vi "Durability_will_2012_07_17_main_single_debug.vi"() -> ()   [LabVIEW 2011]
panel:
  out "error out":errorcluster
  in  "Speed 1":i8(slide)=50 min=0 max=100 step=10 scale=0.0..100.0
  in  "Quit 4":bool
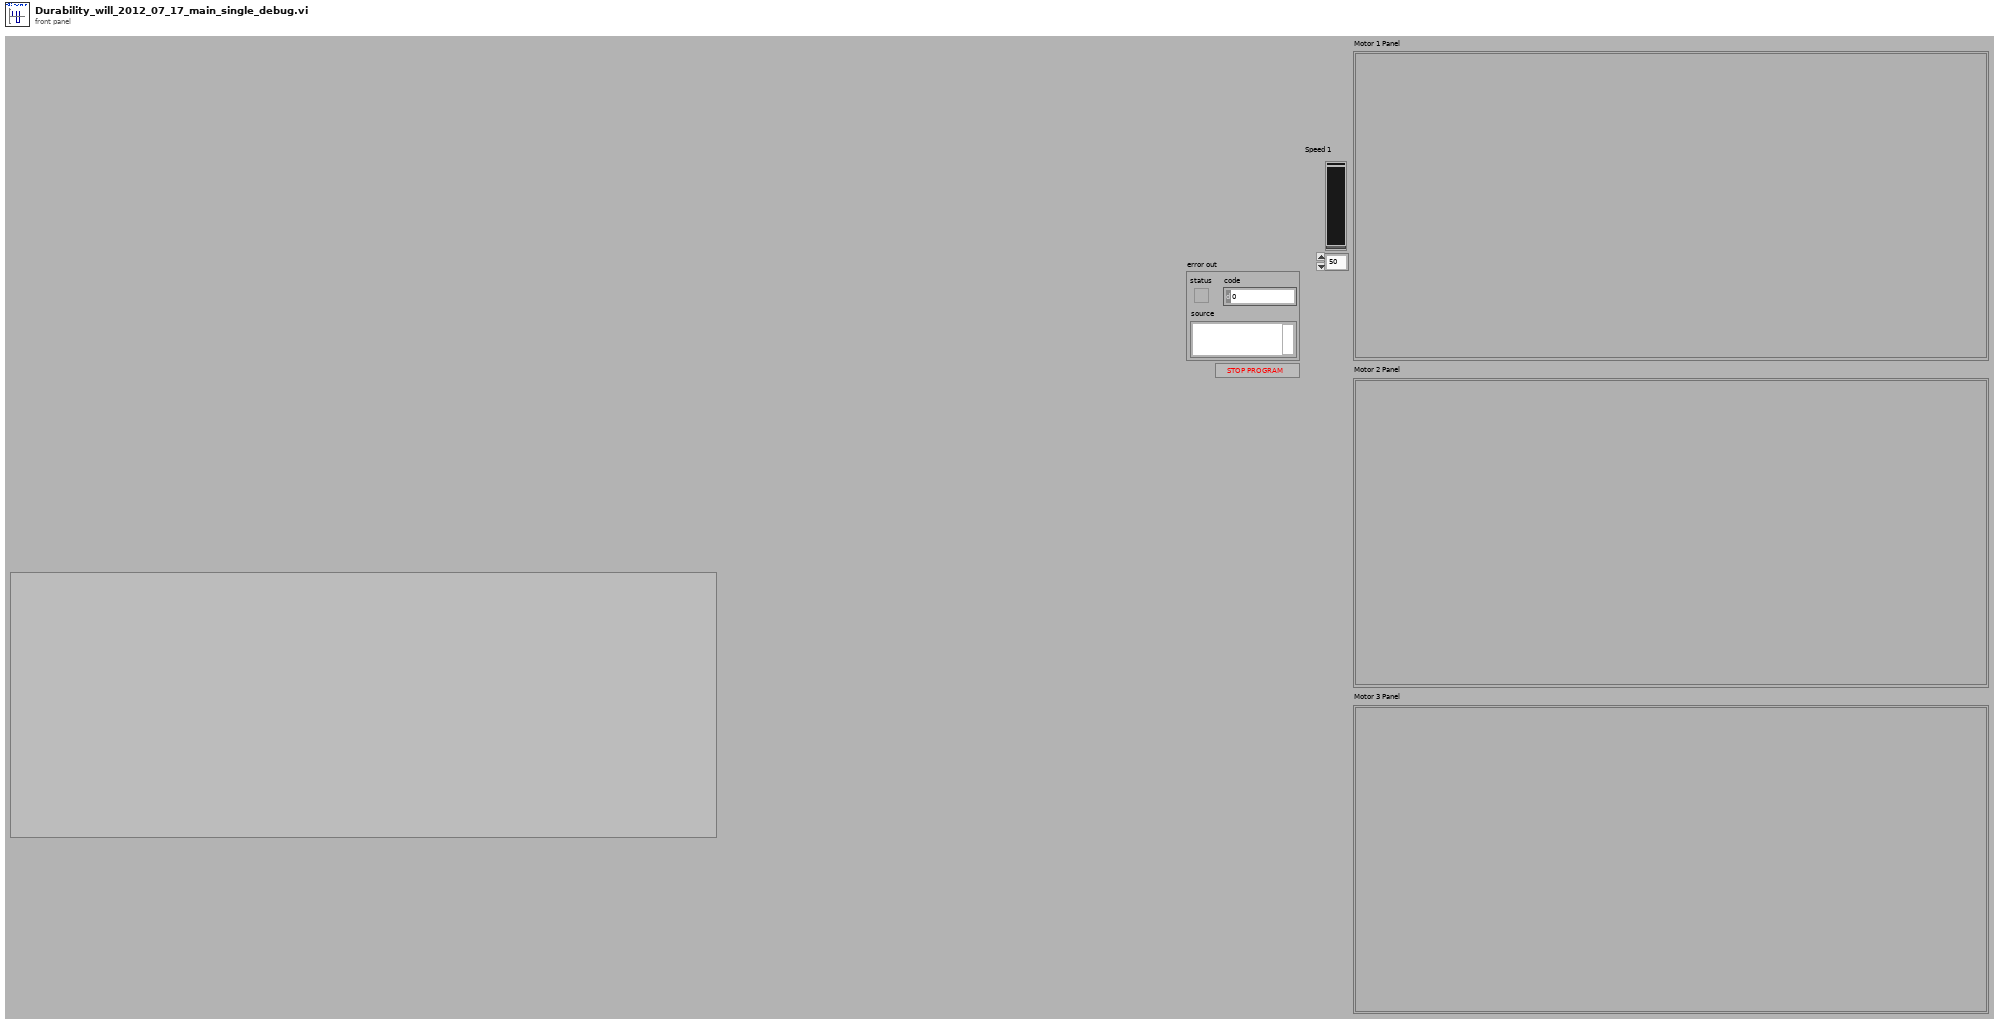
[diagram p1: front panel]
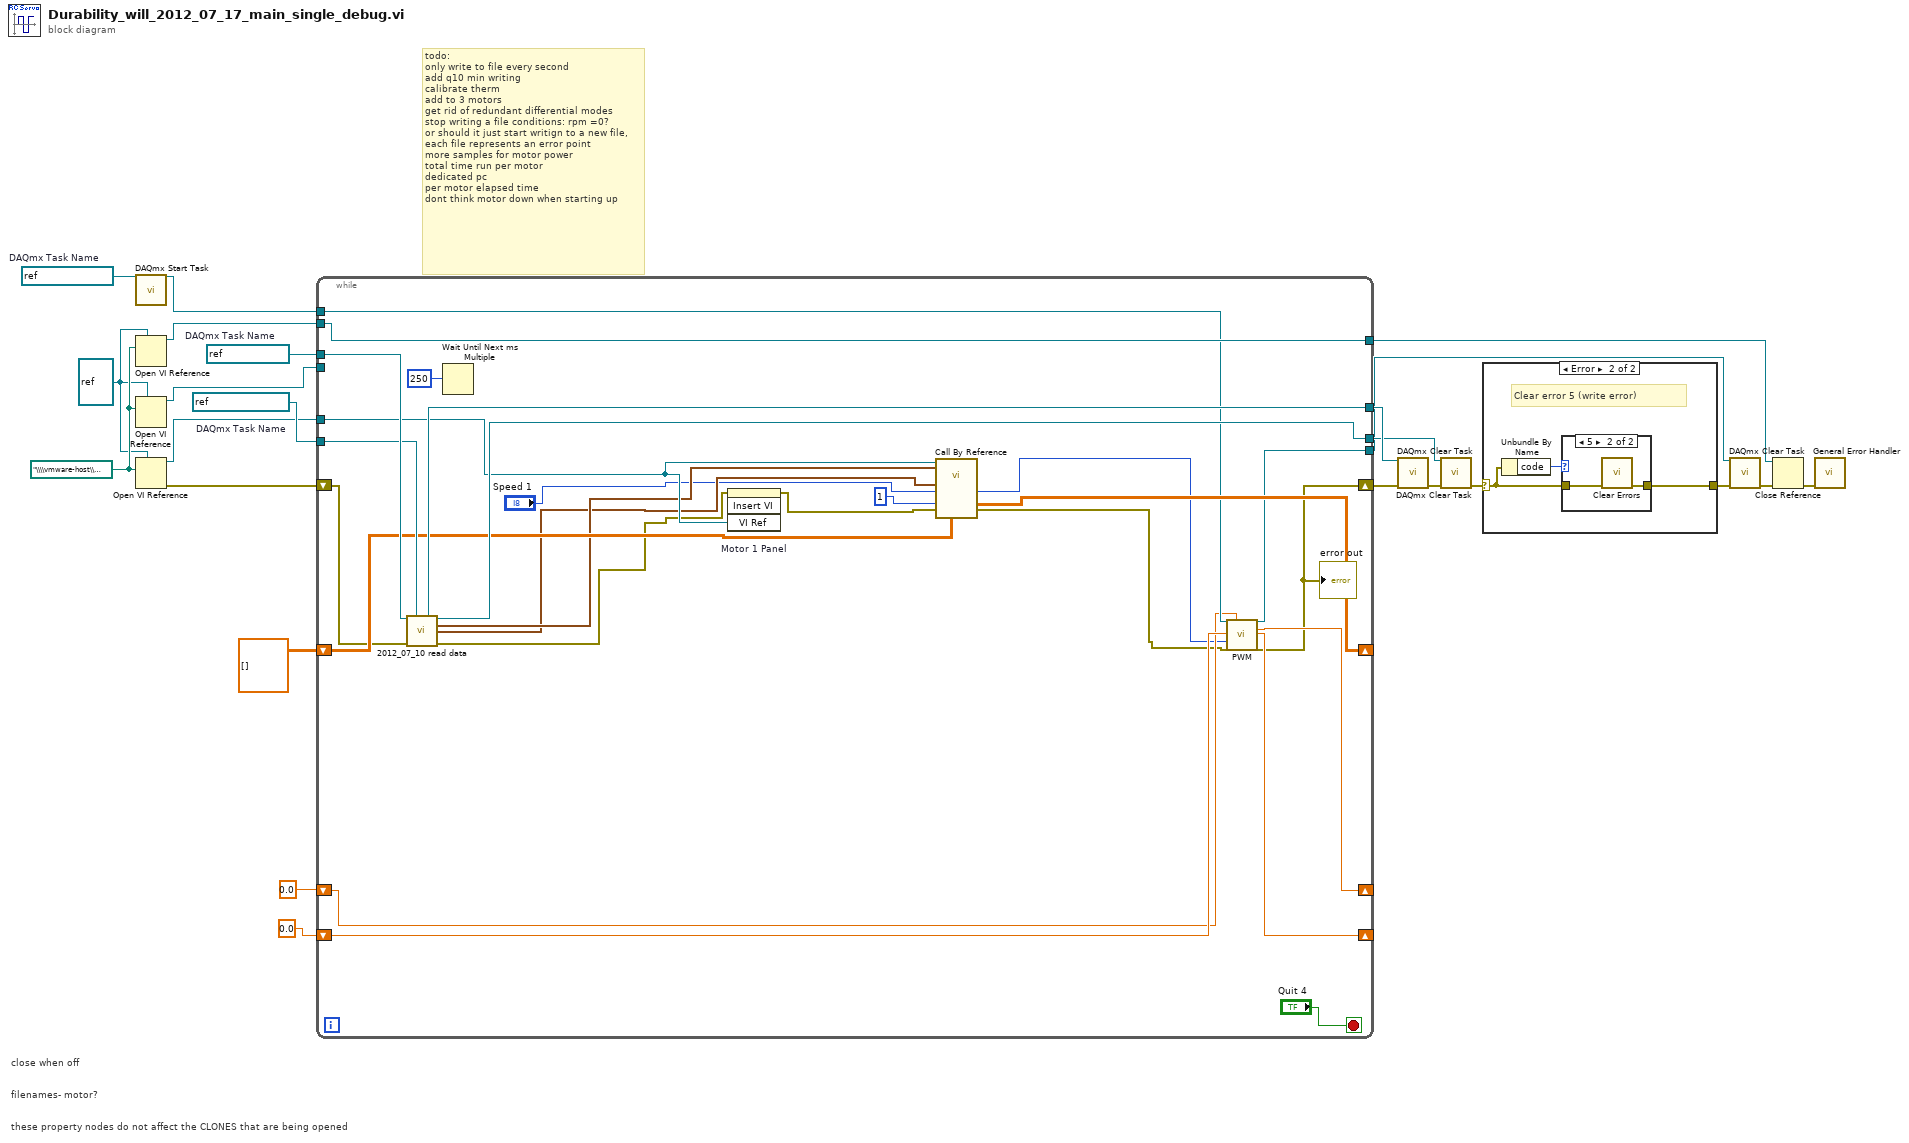
[diagram p0: block diagram]
diagram:
  w5 = refnum<vi> refnum ("type specifier VI Refnum (for type only)")
  w6 = path "\\\\vmware-host\\Shared Folders/wclifton1/Google Drive/Procyrion/Durability/Durability Will/SubVIs/2012_07_10_each motor.vi" ("vi path")
  w9 = refnum<k21> "PWM Signal"  # DAQmx Task Name
  w22 = refnum<k21> "MC Power"  # DAQmx Task Name
  w23 = refnum<k21> "Motor Power"  # DAQmx Task Name
  # "filenames- motor?"
  # "close when off"
  # "these property nodes do not affect the CLONES that are being opened"
  # "todo:\nonly write to file every second\nadd q10 min writing\ncalibrate therm\nadd to 3 motors\nget rid of redundant differential modes\nstop writing a file conditions: rpm =0?\nor should it just start writign to a new file,\neach file represents an error point\nmore samples for motor power\ntotal time run per motor\ndedicated pc\nper motor elapsed time\ndont think motor down when starting up"
  n1 = call <vilib>:"DAQmx Start Task.vi"("task/channels in"=w9) -> ("task out"=w7:refnum<k21>)  [unwired: 13 in, 1 out]
  n2 = Open VI Reference(type specifier VI Refnum (for type only)=w5, vi path=w6) -> (vi reference=w2:refnum<vi>)  [unwired: 4 in, 1 out]
  n3 = Open VI Reference(type specifier VI Refnum (for type only)=w5, vi path=w6) -> (vi reference=w1:refnum<vi>)  [unwired: 4 in, 1 out]
  n4 = Open VI Reference(type specifier VI Refnum (for type only)=w5, vi path=w6) -> (vi reference=w3:refnum<vi>, error out=w8:errorcluster)  [unwired: 4 in]
  n5 = while {
    tunnel: w22 -> [w47]
    tunnel: w23 -> [w46]
    shift-right: [w42] -> _
    shift-left: dbl[][][] [] -> [w43]
    shift-right: [w27] -> w21
    shift-left: w8 -> [w39]
    shift-right: [w31] -> _
    shift-left: 0.0 -> [w32]
    tunnel: [w45] -> w15
    tunnel: [w44] -> w14
    shift-right: [w30] -> _
    shift-left: 0.0 -> [w33]
    tunnel: w3 -> [w41]
    tunnel: [w40] -> w12
    tunnel: w2 -> [w40]
    tunnel: w7 -> [w38]
    tunnel: w1 -> [_]
    tunnel: [w35] -> w4
    stop <- "Quit 4" stop-if-true
    n6 = call "2012_07_10 read data.vi"("MC Power"=w47, "Motor Power"=w46, "Error In"=w39) -> ("Motor Power Out"=w45:refnum<k21>, "MC Power Out"=w44:refnum<k21>, "Motor Power Data"=w37:waveform(dbl)[], "MC Power Data"=w36:waveform(dbl)[], "error out"=w28:errorcluster)  [unwired: 8 in]
    n7 = Wait Until Next ms Multiple(millisecond multiple=u32 250) -> ()  [unwired: 1 out]
    n8 = invoke on="Motor 1 Panel" class="SubPnl" method="Insert VI"(error in=w28, "VI Ref"=w41) -> (error out=w25:errorcluster)  [unwired: 2 in, 3 out]
    n9 = call-by-ref "?"(reference=w41, "MC Power Data In"=w36, "Motor Power Data In"=w37, "Power \nSetting"="Speed 1", "Motor"=i16 1, "Error In"=w25, "Fine Data In"=w43) -> ("Power \nSetting"=w29:i8, "Fine Data Out"=w42:dbl[][][], "Errors"=w24:errorcluster)  [unwired: 8 in, 2 out]
    n10 = call "PWM.vi"("Refnum in"=w38, "High Time In 2"=w33, "Speed 1"=w29, "error in (no error)"=w24, "High Time In 1"=w32) -> ("Refnum out"=w35:refnum<k21>, "High Time Out 1"=w31:dbl, "High Time Out 2"=w30:dbl, "error out"=w27:errorcluster)  [unwired: 19 in]
    "error out" <- w27
  }
  n11 = call <vilib>:"DAQmx Clear Task.vi"("task in"=w15, "error in"=w21) -> ("error out"=w17:errorcluster)  [unwired: 13 in]
  n12 = call <vilib>:"DAQmx Clear Task.vi"("task in"=w14, "error in"=w17) -> ("error out"=w19:errorcluster)  [unwired: 13 in]
  n13 = case shown="Error" w19 {
    selector: w19 -> [w50 w52]
    tunnel: [w50 w51] -> w18
    frame No Error {
    }
    frame Error {
      # "Clear error 5 (write error)"
      n14 = Unbundle By Name(w52) -> ("code"=w53:i32)
      n15 = case shown="5" w53 {
        tunnel: w52 -> [w54 w56]
        tunnel: [w54 w55] -> w51
        frame Default {
        }
        frame 5 {
          n16 = call <vilib>:"Clear Errors.vi"("error in (no error)"=w56) -> ("error out"=w55:errorcluster)  [unwired: 6 in]
        }
      }
    }
  }
  n17 = call <vilib>:"DAQmx Clear Task.vi"("task in"=w4, "error in"=w18) -> ("error out"=w11:errorcluster)  [unwired: 13 in]
  n18 = Close Reference(reference=w12, error in (no error)=w11) -> (error out=w10:errorcluster)
  n19 = call <vilib>:"General Error Handler.vi"("error in (no error)"=w10) -> ()  [unwired: 10 in, 5 out]
